vi "SENSOR_FEATURE_SELECTOR - Type.vi"(8 "error in (no error)":errorcluster) -> (0 "error out":errorcluster, 3 "SENSOR_FEATURE_SELECTOR_VALUE":i32)   [LabVIEW 2013]
doc: "<b>Buffer policy settings can be only unsafe in xiAPI LabVIEW library</b>\nUNSAFE : User gets pointer to internally allocated circle buffer and data may be overwritten by device.\nSAFE : Data from device will be copied to user allocated buffer or xiApi allocated memory."
uses:
  SENSOR_FEATURE_SELECTOR.ctl
  C:/Projects/Cameras3.x/xiLib/xiLIB_64bit/xiLIB/xiCamLib/API/x64/xiApi.NETX64.dll
  xiLIB_64bit/xiLIB/xiCamLib/API/x64/xiApi.NETX64.dll
panel:
  in  "SENSOR_FEATURE_SELECTOR":T1
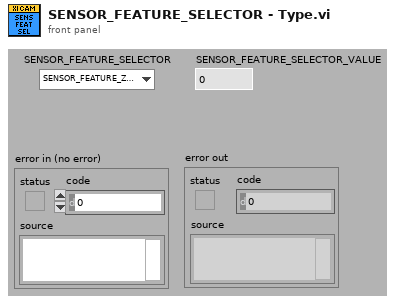
[diagram p1: front panel]
types:
  T1 = typedef "SENSOR_FEATURE_SELECTOR.ctl" = enum16{"SENSOR_FEATURE_ZEROROT_ENABLE"}
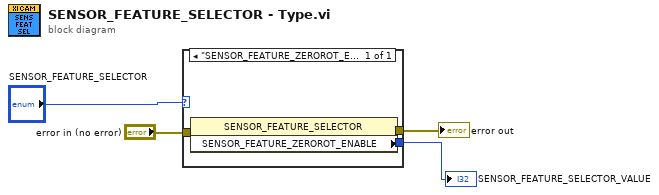
[diagram p0: block diagram]
diagram:
  n1 = case shown="\"SENSOR_FEATURE_ZEROROT_ENABLE\"" "SENSOR_FEATURE_SELECTOR" {
    tunnel: "error in (no error)" -> [w7]
    tunnel: [w6] -> w3
    tunnel: [w5] -> w2
    frame "SENSOR_FEATURE_ZEROROT_ENABLE" {
      n2 = property class="SENSOR_FEATURE_SELECTOR"(error in=w7) -> (error out=w6:errorcluster, "SENSOR_FEATURE_ZEROROT_ENABLE"=w5:i32)  [unwired: 1 in, 1 out]
    }
  }
  "error out" <- w3
  "SENSOR_FEATURE_SELECTOR_VALUE" <- w2
